vi "Setup.vi"(11 "Dev Panel in":refnum<class "Dev Panel.lvclass">) -> (0 "error out":errorcluster, 3 "Dev Panel out":refnum<class "Dev Panel.lvclass">)   [LabVIEW 2021, in "Dev Panel.lvclass"]
uses:
  Dev Panel.lvclass
  Dev Panel.lvclass/Dev Panel.ctl
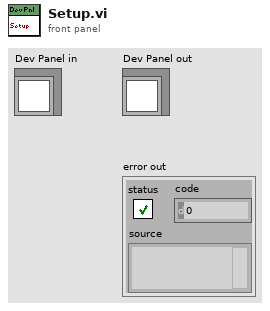
[diagram p1: front panel]
types:
  T1 = enum32{"Invalid", "Standard", "Closed", "Hidden", "Minimized", "Maximized"}
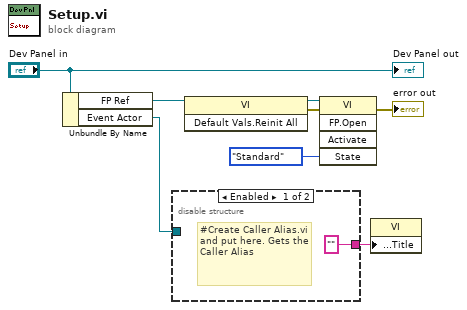
[diagram p0: block diagram]
diagram:
  n1 = Unbundle By Name("Dev Panel in") -> ("FP Ref"=w3:refnum<vi>, "Event Actor"=w1:refnum<class "Event Actor.lvclass">)
  n2 = disable-structure shown="Enabled" {
    disable-tunnel: ["" ("Front Panel Window:Title") _] -> w2
    disable-tunnel: w1 -> [_ _]
    frame Enabled {
      # "#Create Caller Alias.vi\nand put here. Gets the Caller Alias"
    }
    frame Disabled {
    }
  }
  n3 = invoke class="VI" method="Default Vals.Reinit All"(reference=w3) -> (reference out=w4:refnum<vi>, error out=w5:errorcluster)  [unwired: 2 in, 1 out]
  n4 = invoke class="VI" method="FP.Open"(reference=w4, error in=w5, "State"=T1."Standard") -> (error out=→"error out":errorcluster)  [unwired: 2 in, 4 out]
  n5 = property class="VI"("Front Panel.Title"=w2) -> ()  [unwired: 2 in, 2 out]
  "Dev Panel out" <- "Dev Panel in"
